vi "Buffer Command Log.vi"() -> (2 "File Reference Out":refnum<file>)   [LabVIEW 2016]
uses:
  Global Variables/Folder Names.vi
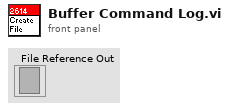
[diagram p1: front panel]
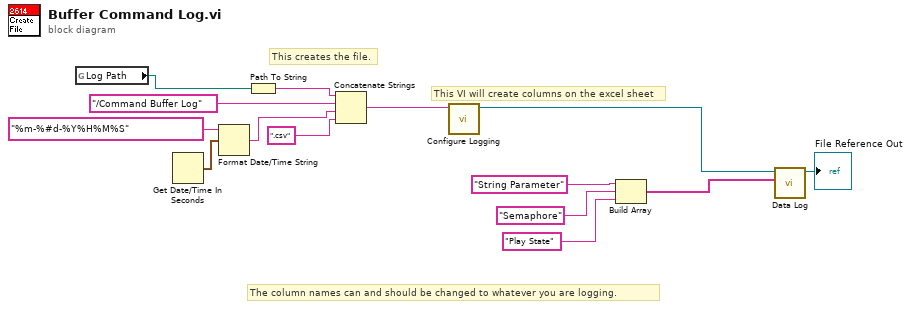
[diagram p0: block diagram]
diagram:
  # "The column names can and should be changed to whatever you are logging."
  # "This VI will create columns on the excel sheet"
  # "This creates the file."
  n1 = global read "Folder Names.vi" "Log Path"() -> (w12:path)
  n2 = Get Date/Time In Seconds() -> (seconds since 1Jan1904=w7:timestamp)
  n3 = Format Date/Time String(time format string (%c)="%m-%#d-%Y%H%M%S", seconds (now)=w7) -> (date/time string=w5:string)  [unwired: 1 in]
  n4 = Path To String(path=w12) -> (string=w11:string)
  n5 = Concatenate Strings(w11, "/Command Buffer Log" ("string"), w5, ".csv" ("string")) -> (w13:string)
  n6 = call "Configure Logging.vi"("File Path/File Name"=w13) -> ("refnum out"=w9:refnum<file>)  [unwired: 10 in]
  n7 = Build Array("String Parameter" ("File Path/File Name"), "Semaphore" ("File Path/File Name"), "Play State" ("element")) -> (w10:string[])
  n8 = call "Data Log.vi"("Data In"=w10, "File Reference In"=w9) -> ("File Reference Out"=→"File Reference Out":refnum<file>)  [unwired: 9 in]
